vi "FormVarValuesArray.vi"(2 "varables bytes":i32[](array[numeric]), 3 "varables ports":i32[](array[numeric]), 4 "Ports":u8[](array[numeric])) -> (1 "Values Array":string[](array[string]))   [LabVIEW 2010]
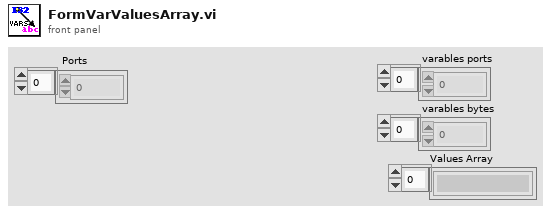
[diagram p1: front panel]
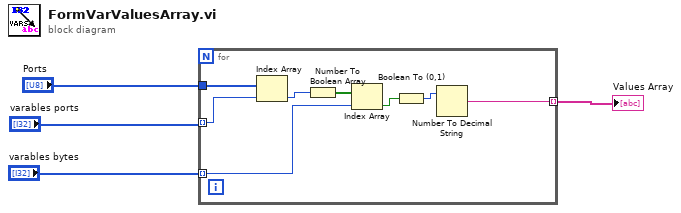
[diagram p0: block diagram]
diagram:
  n1 = for {
    tunnel: "varables ports" -> [w11] mode=indexing
    tunnel: "Ports" -> [w12]
    tunnel: "varables bytes" -> [w8] mode=indexing
    tunnel: [w5] -> w1 mode=indexing
    n2 = Index Array(array=w12, index=w11) -> (element=w10:u8)
    n3 = Number To Boolean Array(number=w10) -> (Boolean array=w9:bool[])
    n4 = Index Array(array=w9, index=w8) -> (element=w7:bool)
    n5 = Boolean To (0,1)(Boolean=w7) -> (0, 1=w6:i16)
    n6 = Number To Decimal String(number=w6) -> (decimal integer string=w5:string)  [unwired: 1 in]
  }
  "Values Array" <- w1
